vi "Blink 6 shift refs.vi"(8 "Error In":errorcluster) -> (0 "Error Out":errorcluster)   [LabVIEW 2014]
uses:
  <vilib>/Aledyne-TSXperts/Arduino Compatible Compiler for LabVIEW/addons/Arduino SoftwareSerial Wrapper/Arduino SoftwareSerial Wrapper.lvlib
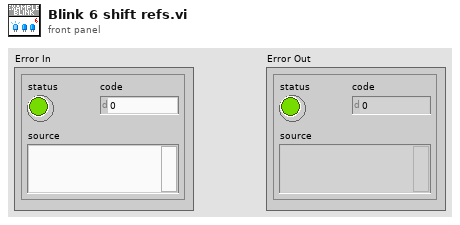
[diagram p1: front panel]
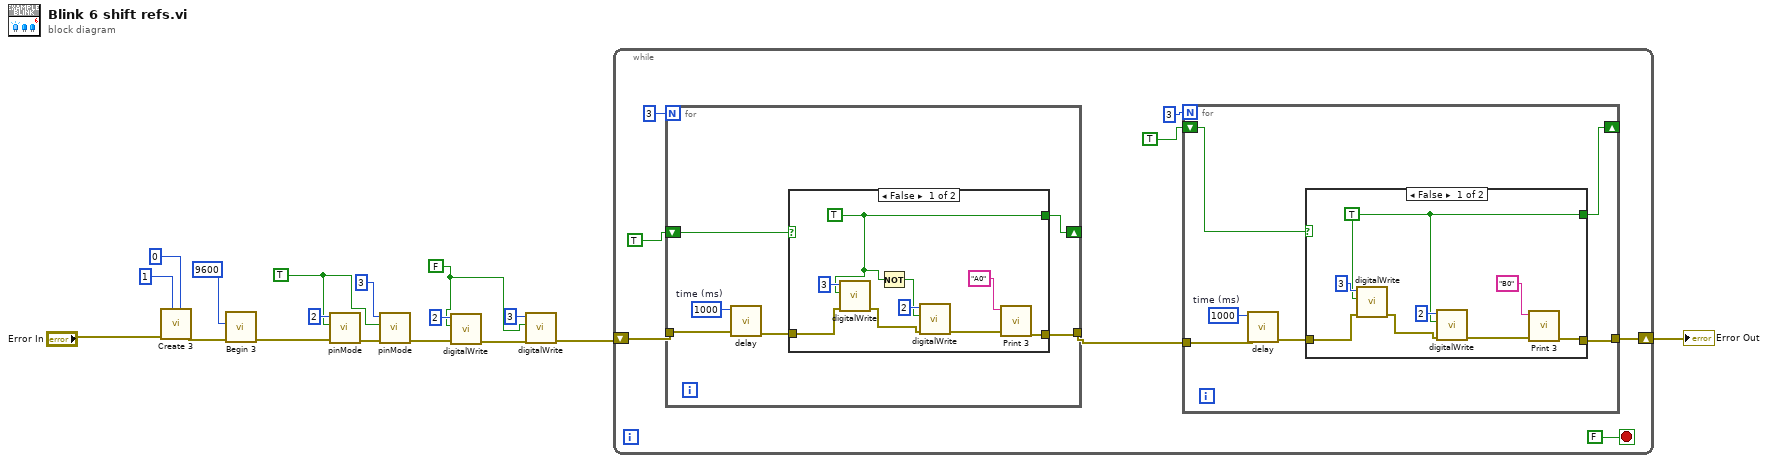
[diagram p0: block diagram]
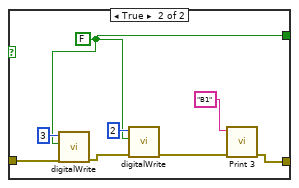
[diagram p2: hidden frame]
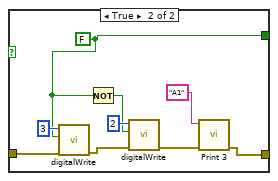
[diagram p3: hidden frame]
diagram:
  w7 = FALSE
  w14 = TRUE
  n1 = call <vilib>:"Create 3.vi"("arduino RX pin"=u8 0, "arduino TX pin"=u8 1, "Error In"="Error In") -> ("Error Out"=w4:errorcluster)  [unwired: 8 in]
  n2 = call <vilib>:"Begin 3.vi"("Error In"=w4, "Baudrate"=u16 9600) -> ("Error Out"=w2:errorcluster)  [unwired: 8 in]
  n3 = call "pinMode.vi"("Error In"=w2, "output?"=w14, "pin number"=2) -> ("Error Out"=w17:errorcluster)  [unwired: 8 in]
  n4 = call "pinMode.vi"("Error In"=w17, "output?"=w14, "pin number"=3) -> ("Error Out"=w10:errorcluster)  [unwired: 8 in]
  n5 = call "digitalWrite.vi"("Error In"=w10, "value"=w7, "pin number"=2) -> ("Error Out"=w9:errorcluster)  [unwired: 8 in]
  n6 = call "digitalWrite.vi"("Error In"=w9, "value"=w7, "pin number"=3) -> ("Error Out"=w8:errorcluster)  [unwired: 8 in]
  n7 = while {
    shift-right: [w22] -> w13
    shift-left: w8 -> [w25]
    stop <- FALSE stop-if-true
    n8 = for {
      N: 3 -> [_]
      tunnel: w25 -> [w53]
      tunnel: [w50] -> w20
      shift-right: [w48] -> _
      shift-left: TRUE -> [w49]
      w51 = 1000  # time (ms)
      n9 = call "delay.vi"("Error In"=w53, "time (ms)"=w51) -> ("Error Out"=w52:errorcluster)  [unwired: 9 in]
      n10 = case shown="False" w49 {
        tunnel: w52 -> [w61 w71]
        tunnel: [w54 w64] -> w50
        tunnel: [w58 w67] -> w48
        frame False {
          w58 = TRUE
          n11 = call "digitalWrite.vi"("Error In"=w61, "value"=w58, "pin number"=3) -> ("Error Out"=w57:errorcluster)  [unwired: 8 in]
          n12 = Not(x=w58) -> (.not. x?=w59:bool)
          n13 = call "digitalWrite.vi"("Error In"=w57, "value"=w59, "pin number"=2) -> ("Error Out"=w55:errorcluster)  [unwired: 8 in]
          n14 = call <vilib>:"Print 3.vi"("Error In"=w55, "String to print"="A0") -> ("Error Out"=w54:errorcluster)  [unwired: 9 in]
        }
        frame True {
          w67 = FALSE
          n15 = call "digitalWrite.vi"("Error In"=w71, "value"=w67, "pin number"=3) -> ("Error Out"=w68:errorcluster)  [unwired: 8 in]
          n16 = Not(x=w67) -> (.not. x?=w66:bool)
          n17 = call "digitalWrite.vi"("Error In"=w68, "value"=w66, "pin number"=2) -> ("Error Out"=w65:errorcluster)  [unwired: 8 in]
          n18 = call <vilib>:"Print 3.vi"("Error In"=w65, "String to print"="A1") -> ("Error Out"=w64:errorcluster)  [unwired: 9 in]
        }
      }
    }
    n19 = for {
      N: 3 -> [_]
      tunnel: [w29] -> w22
      tunnel: w20 -> [w28]
      shift-right: [w26] -> _
      shift-left: TRUE -> [w27]
      w30 = 1000  # time (ms)
      n20 = call "delay.vi"("Error In"=w28, "time (ms)"=w30) -> ("Error Out"=w31:errorcluster)  [unwired: 9 in]
      n21 = case shown="False" w27 {
        tunnel: w31 -> [w38 w47]
        tunnel: [w32 w40] -> w29
        tunnel: [w36 w43] -> w26
        frame False {
          w36 = TRUE
          n22 = call "digitalWrite.vi"("Error In"=w38, "value"=w36, "pin number"=3) -> ("Error Out"=w35:errorcluster)  [unwired: 8 in]
          n23 = call "digitalWrite.vi"("Error In"=w35, "value"=w36, "pin number"=2) -> ("Error Out"=w33:errorcluster)  [unwired: 8 in]
          n24 = call <vilib>:"Print 3.vi"("Error In"=w33, "String to print"="B0") -> ("Error Out"=w32:errorcluster)  [unwired: 9 in]
        }
        frame True {
          w43 = FALSE
          n25 = call "digitalWrite.vi"("Error In"=w47, "value"=w43, "pin number"=3) -> ("Error Out"=w44:errorcluster)  [unwired: 8 in]
          n26 = call "digitalWrite.vi"("Error In"=w44, "value"=w43, "pin number"=2) -> ("Error Out"=w41:errorcluster)  [unwired: 8 in]
          n27 = call <vilib>:"Print 3.vi"("Error In"=w41, "String to print"="B1") -> ("Error Out"=w40:errorcluster)  [unwired: 9 in]
        }
      }
    }
  }
  "Error Out" <- w13
